vi "34461A.vi"() -> ()   [LabVIEW 2014]
uses:
  <instrlib>/Agilent 3446X Series/Public/Data/Read (Single Point).vi
  <instrlib>/Agilent 3446X Series/Agilent 3446X Series.lvlib
panel:
  in  "Manual Range":dbl=10.0
  out "波形图表":dbl[](graph)
  in  "Sample Period(ms)":dbl=100.0
  out "已采样数量":dbl
  in  "Data Collection Switch":bool
  in  "Aperture Time":sgl(ring)=1.0 items=["100"=100, "10"=10, "1"=1, "0.2"=0.2, "0.02"=0.02]
  in  "Auto Zero":enum16{"Off", "On"}(ring)=enum."On"
  in  "VISA resource name":refnum<visa-resource-name>
  in  "Auto Range":bool=TRUE
  in  "Absolute Resolution":dbl=1e-06
  in  "Measurement Function":i32(ring)=10 items=["Continuity", "Current AC", "Current DC", "Diode", "Frequency", "Resistance 4-wire", "Period", "Resistance 2-wire", "Temperature", "Voltage AC", "Voltage DC", "Voltage DC Ratio"]
  in  "路径":path=path "data"
  # "Note：before running the program ,open the Data Collection Switch .Use the Data Collection Switch to stop the program."
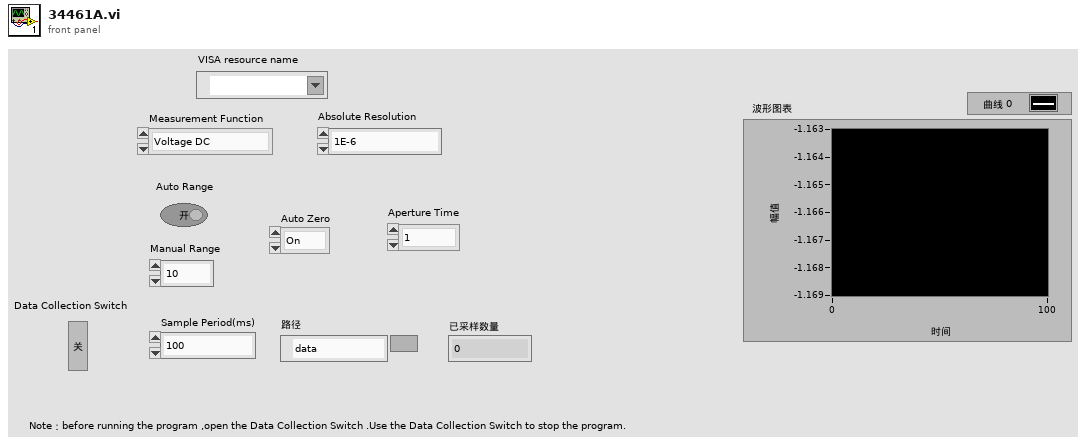
[diagram p1: front panel]
types:
  T1 = enum16{"open", "open or create", "create or replace", "create", "open (read-only)"}
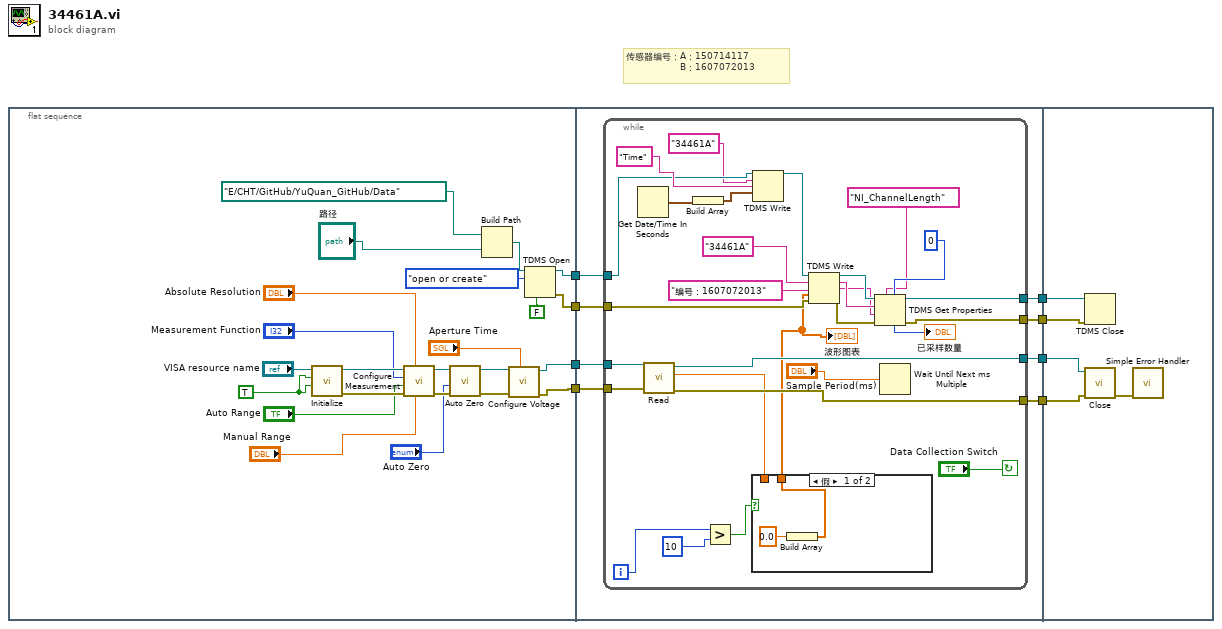
[diagram p0: block diagram]
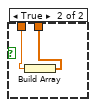
[diagram p2: hidden frame]
diagram:
  # "传感器编号：A：150714117\n                  B：1607072013"
  n1 = flat-sequence {
    tunnel: [w10] -> w8
    tunnel: [w9] -> w7
    tunnel: [w18] -> w6
    tunnel: [w17] -> w2
    tunnel: w8 -> [w38]
    tunnel: w7 -> [w37]
    tunnel: w6 -> [w39]
    tunnel: [w36] -> w5
    tunnel: [w35] -> w4
    tunnel: [w34] -> w3
    tunnel: w2 -> [w33]
    tunnel: [w32] -> w1
    tunnel: w5 -> [w76]
    tunnel: w4 -> [w75]
    tunnel: w3 -> [w74]
    tunnel: w1 -> [w73]
    frame #0 {
      w16 = TRUE
      n2 = call <instrlib>:"Initialize.vi"("Reset (True)"=w16, "ID Query (True)"=w16, "VISA resource name"="VISA resource name") -> ("error out"=w25:errorcluster, "VISA resource name out"=w26:refnum<visa-resource-name>)  [unwired: 2 in, 5 out]
      n3 = call <instrlib>:"Configure Measurement.vi"("Manual Range (1)"="Manual Range", "Absolute Resolution (1E-6)"="Absolute Resolution", "error in (no error)"=w25, "Auto Range (T: Enable)"="Auto Range", "Measurement Function (10: Voltage DC)"="Measurement Function", "VISA resource name"=w26) -> ("error out"=w20:errorcluster, "VISA resource name out"=w19:refnum<visa-resource-name>)  [unwired: 4 out]
      n4 = call <instrlib>:"Auto Zero.vi"("error in (no error)"=w20, "Auto Zero (1: Enable)"="Auto Zero", "VISA resource name"=w19) -> ("error out"=w12:errorcluster, "VISA resource name out"=w13:refnum<visa-resource-name>)  [unwired: 7 in]
      n5 = Build Path(base path=path "E:/CHT/GitHub/YuQuan_GitHub/Data", name or relative path="路径") -> (appended path=w30:path)
      n6 = call <instrlib>:"Configure Voltage.vi"("Voltage Integration Time (10: 10)"="Aperture Time", "error in (no error)"=w12, "VISA resource name"=w13) -> ("error out"=w9:errorcluster, "VISA resource name out"=w10:refnum<visa-resource-name>)  [unwired: 7 in]
      n7 = TDMS Open(6:FALSE ("disable buffering (T)"), 10:T1."open or create" ("operation"), 11:w30) -> (0:w17:errorcluster, 3:w18:refnum<k34>)  [unwired: 4 in]
    }
    frame #1 {
      n8 = while {
        tunnel: w39 -> [w50]
        tunnel: w38 -> [w43]
        tunnel: w37 -> [w42]
        tunnel: [w60] -> w36
        tunnel: [w59] -> w35
        tunnel: [w58] -> w34
        tunnel: w33 -> [w57]
        tunnel: [w55] -> w32
        i -> [w47]
        stop <- "Data Collection Switch" continue-if-true
        n9 = Get Date/Time In Seconds() -> (seconds since 1Jan1904=w53:timestamp)
        n10 = call-poly <instrlib>:"Read.vi"("error in (no error)"=w42, "VISA resource name"=w43) -> ("error out"=w59:errorcluster, "Measurement"=w41:dbl, "VISA resource name out"=w60:refnum<visa-resource-name>)  [unwired: 1 in, 6 out]
        n11 = Build Array(w53) -> (w52:timestamp[])
        n12 = Greater?(x=w47, y=10) -> (0:w45:bool)
        n13 = case shown="假" w45 {
          tunnel: w41 -> [_ w72]
          tunnel: [w69 w71] -> w40
          frame False {
            n14 = Build Array(0.0) -> (w69:dbl[])
          }
          frame True {
            n15 = Build Array(w72) -> (w71:dbl[])
          }
        }
        "波形图表" <- w40
        n16 = TDMS Write(0:w50, 5:"34461A", 7:"Time", 9:w52) -> (4:w49:refnum<k34>)  [unwired: 2 in, 3 out]
        n17 = TDMS Write(0:w49, 5:"34461A", 7:"编号：1607072013", 9:w40, 11:w57) -> (4:w65:refnum<k34>, 6:w64:string, 8:w63:string, 15:w56:errorcluster)  [unwired: 1 in]
        n18 = TDMS Get Properties(5:0, 7:"NI_ChannelLength", 8:w56, 9:w63, 10:w64, 11:w65) -> (0:w55:errorcluster, 3:w58:refnum<k34>, 4:→"已采样数量":i32)  [unwired: 3 out]
        n19 = Wait Until Next ms Multiple(millisecond multiple="Sample Period(ms)") -> ()  [unwired: 1 out]
      }
    }
    frame #2 {
      n20 = TDMS Close(8:w73, 11:w74) -> ()  [unwired: 2 out]
      n21 = call <instrlib>:"Close.vi"("error in (no error)"=w75, "VISA resource name"=w76) -> ("error out"=w77:errorcluster)  [unwired: 9 out]
      n22 = call <vilib>:"Simple Error Handler.vi"("error in (no error)"=w77) -> ()  [unwired: 1 in, 8 out]
    }
  }
